vi "UDP Factory.vi"(8 "error in (no error)":errorcluster, 10 "UDP Settings":T1) -> (0 "error out":errorcluster, 3 "UDP out":refnum<class "UDP.lvclass">)   [LabVIEW 2019, in "Protocols.lvlib" / "UDP.lvclass"]
uses:
  UDP.lvclass
  Control 4.ctl
  UDP.lvclass/UDP.ctl
  Data Access/Write Local IP Address.vi
  Data Access/Write Local Port.vi
  Data Access/Write Target IP Address.vi
  Data Access/Write Target Port.vi
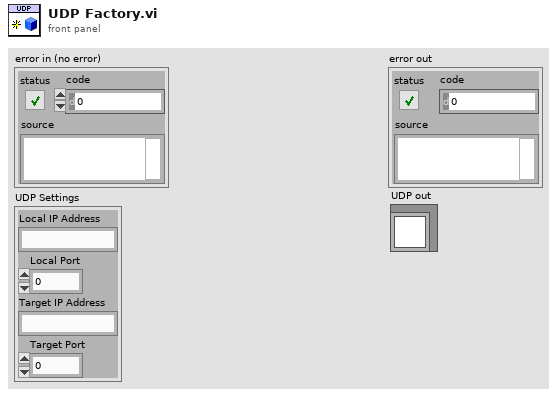
[diagram p1: front panel]
types:
  T1 = typedef "Control 4.ctl" = cluster{"Local IP Address":string, "Local Port":u16, "Target IP Address":string, "Target Port":u16}
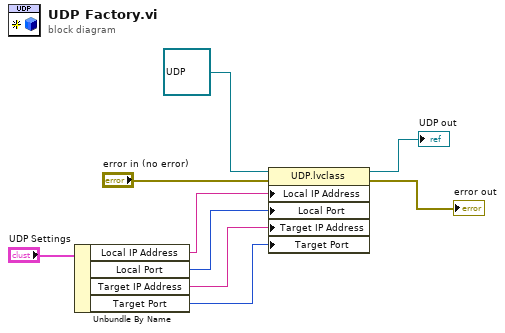
[diagram p0: block diagram]
diagram:
  n1 = Unbundle By Name("UDP Settings") -> ("Local IP Address"=w4:string, "Local Port"=w3:u16, "Target IP Address"=w2:string, "Target Port"=w1:u16)
  n2 = property class="UDP.lvclass"(reference=refnum<class "UDP.lvclass"> refnum ("Protocols.lvlib:UDP.lvclass"), error in="error in (no error)", "Local IP Address"=w4, "Local Port"=w3, "Target IP Address"=w2, "Target Port"=w1) -> (reference out=→"UDP out":refnum<class "UDP.lvclass">, error out=→"error out":errorcluster)
